vi "Write Waveform.vi"(8 "error in (no error)":errorcluster, 10 "Waveform":waveform(dbl)[](array[waveform]), 11 "Linear_Task in":refnum<class "Linear_Task.lvclass">) -> (0 "error out":errorcluster, 3 "Linear_Task out":refnum<class "Linear_Task.lvclass">)   [LabVIEW 2025, in "Linear_Task.lvlib" / "Linear_Task.lvclass"]
uses:
  Linear_Task.lvclass
  Linear_Task.lvclass/Linear_Task.ctl
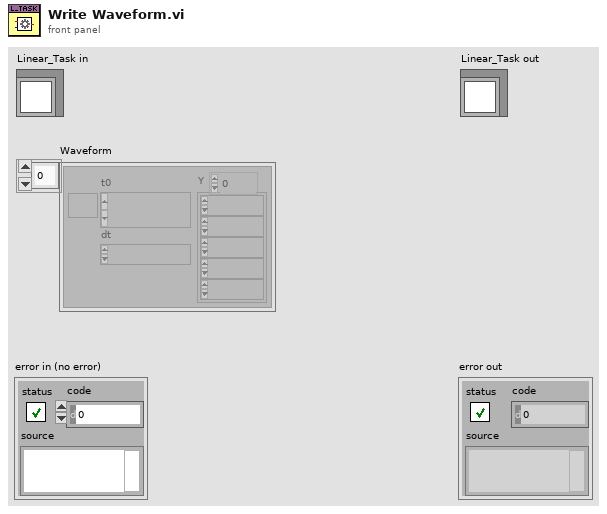
[diagram p1: front panel]
types:
  T1 = typedef "Task_Abstr.lvlib/Task_Abstr.lvclass/DataContainer.ctl" = map{string, T2}
  T2 = typedef "Task_Abstr.lvlib/Task_Abstr.lvclass/WaveformData.ctl" = cluster{"StartTime":timestamp, "StopTime":timestamp, "Waveform":waveform(dbl)[]}
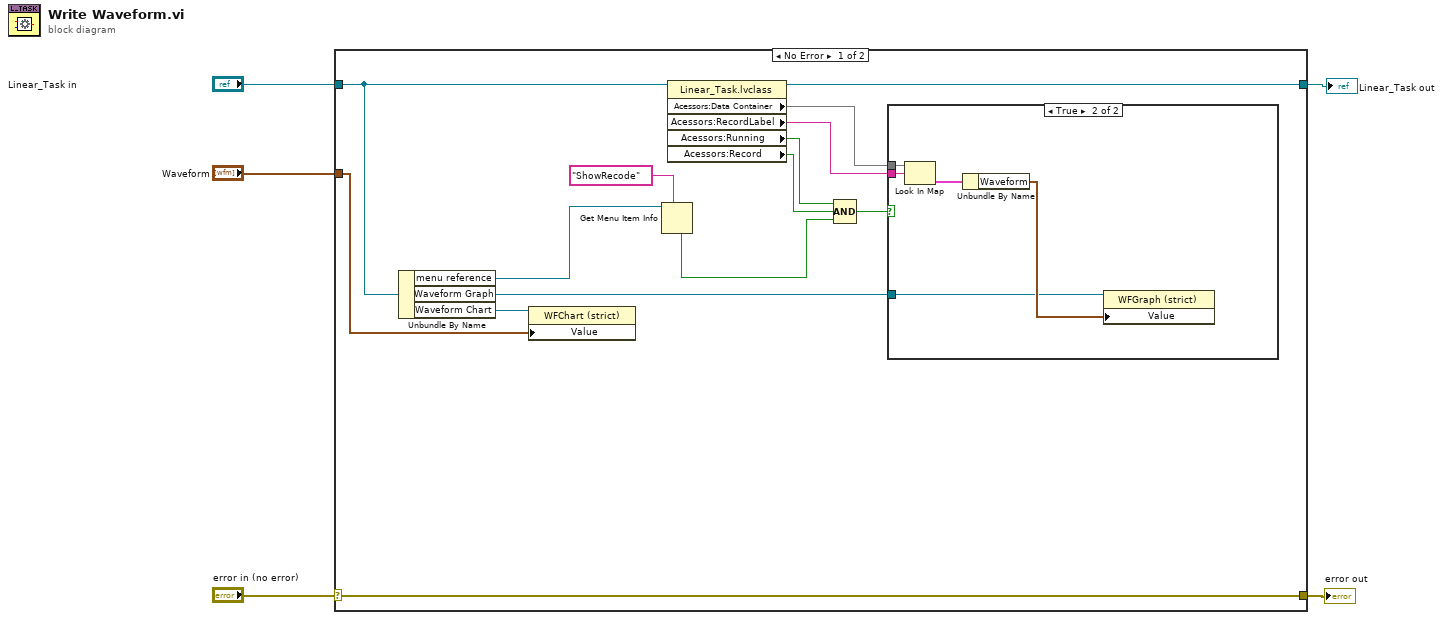
[diagram p0: block diagram]
diagram:
  n1 = case shown="No Error" "error in (no error)" {
    selector: "error in (no error)" -> [w19 w25]
    tunnel: [w19 w25] -> w4
    tunnel: [w6 w26] -> w2
    tunnel: "Linear_Task in" -> [w8 w26]
    tunnel: "Waveform" -> [w7 _]
    frame No Error {
      n2 = Unbundle By Name(w8) -> ("menu reference"=w12:refnum<k9>, "Waveform Graph"=w15:refnum<vi>, "Waveform Chart"=w18:refnum<vi>)
      n3 = property class="WFChart (strict)"(reference=w18, "Value"=w7) -> ()  [unwired: 1 in, 2 out]
      n4 = Get Menu Item Info(7:"ShowRecode" ("item tag"), 11:w12) -> (4:w10:bool)  [unwired: 1 in, 6 out]
      n5 = property class="Linear_Task.lvclass"(reference=w8) -> (reference out=w6:refnum<class "Linear_Task.lvclass">, "Acessors:Data Container"=w17:T1, "Acessors:RecordLabel"=w16:string, "Acessors:Running"=w14:bool, "Acessors:Record"=w13:bool)  [unwired: 1 in, 1 out]
      n6 = Compound Arithmetic op=AND(w14, w13, w10) -> (w9:bool)
      n7 = case shown="True" w9 {
        tunnel: w17 -> [_ w24]
        tunnel: w16 -> [_ w23]
        tunnel: w15 -> [_ w20]
        frame False {
        }
        frame True {
          n8 = Look In Map(map=w24, key=w23) -> (value=w22:T2)  [unwired: 1 in, 1 out]
          n9 = Unbundle By Name(w22) -> ("Waveform"=w21:waveform(dbl)[])
          n10 = property class="WFGraph (strict)"(reference=w20, "Value"=w21) -> ()  [unwired: 1 in, 2 out]
        }
      }
    }
    frame Error {
    }
  }
  "error out" <- w4
  "Linear_Task out" <- w2
